vi "Frequency Amplitude Stepped Sweep.vi"(0 "Semiconductor Module Context":T2, 1 "Frequency Sweep (Hz)":dbl[](array[numeric]), 2 "Amplitude Sweep (V)":dbl[](array[numeric]), 5 "Ref Mic Sampling Rate (Hz)":dbl format="%#_13g", 7 "Speaker Sampling Rate (Hz)":dbl format="%#_13g", 11 "error in (no error)":errorcluster) -> (4 "Per-Site Per-Freq Per-Amp dB SPL":dbl[][][](array[numeric]), 15 "error out":errorcluster)   [LabVIEW 2020]
doc: "Frequency Amplitude Stepped Sweep VI returns the Per-Site dB SPL array obtained by sweeping over frequency and amplitude. Also, this VI provides Per-Site TED Bitstream for the passed TSM reference."
uses:
  <vilib>/NI_TestStand_SemiconductorModule/NI_TestStand_Semiconductor_Module.lvlibp/PinMap/General/SemiconductorModuleContext.ctl
  e4dca00a-4e93-4fe6-a22a-85184fe6c6d7.vi
  6f0c4c81-6e94-4ac5-a946-327ae8ed193a.vi
  66372b91-0235-4dd9-a3ee-ceaa2015ee1b.vi
  <vilib>/measure/matone.llb/Extract Single Tone Information N Chan.vi
  <vilib>/NI_TestStand_SemiconductorModule/NI_TestStand_Semiconductor_Module.lvlibp
  <vilib>/measure/NI_MAPro.lvlib
panel:
  in  "Abort":bool
  out "Calibration Progress":dbl(slide) scale=0.0..1.0
  out "Speaker Amplitude":T1(slide)={"Numeric"=0.001, "Numeric"=1.0, "Numeric"=0.001} scale=0.0001..10.0 scale format="%#_6pV"
  out "Frequency":T1(slide)={"Numeric"=100.0, "Numeric"=20000.0, "Numeric"=100.0} scale=10.0..100000.0 scale format="%#_6pHz"
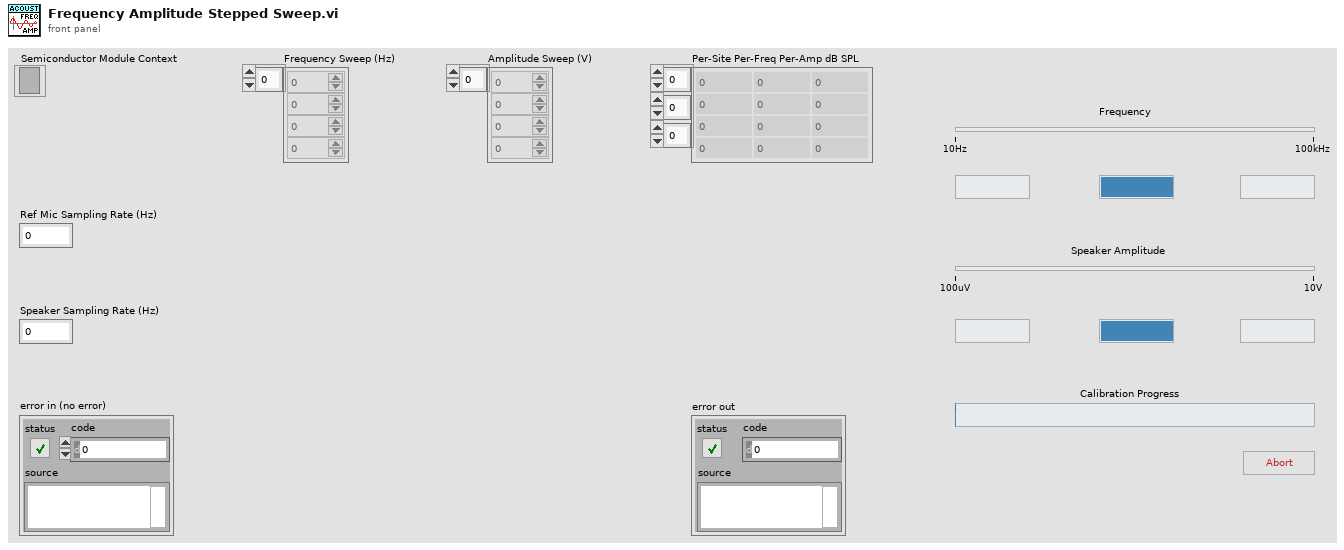
[diagram p1: front panel]
types:
  T1 = cluster{"Numeric":dbl, "Numeric":dbl, "Numeric":dbl}
  T2 = typedef "NI_TestStand_Semiconductor_Module.lvlibp/SemiconductorModuleContext.ctl" = refnum<k7>
  T3 = typedef "TSM DAQmx Multi-Task.ctl" = cluster{"Pin Query Context":refnum<class "MultiplePinMultipleSessionQueryContext.lvclass">, "SSC":T4[], "Site Numbers":i32[], "Pins":tag[]}
  T4 = typedef "SSC DAQmx.ctl" = cluster{"DAQmx Task ":refnum<k21>, "Channels":string, "Channel Lists":string}
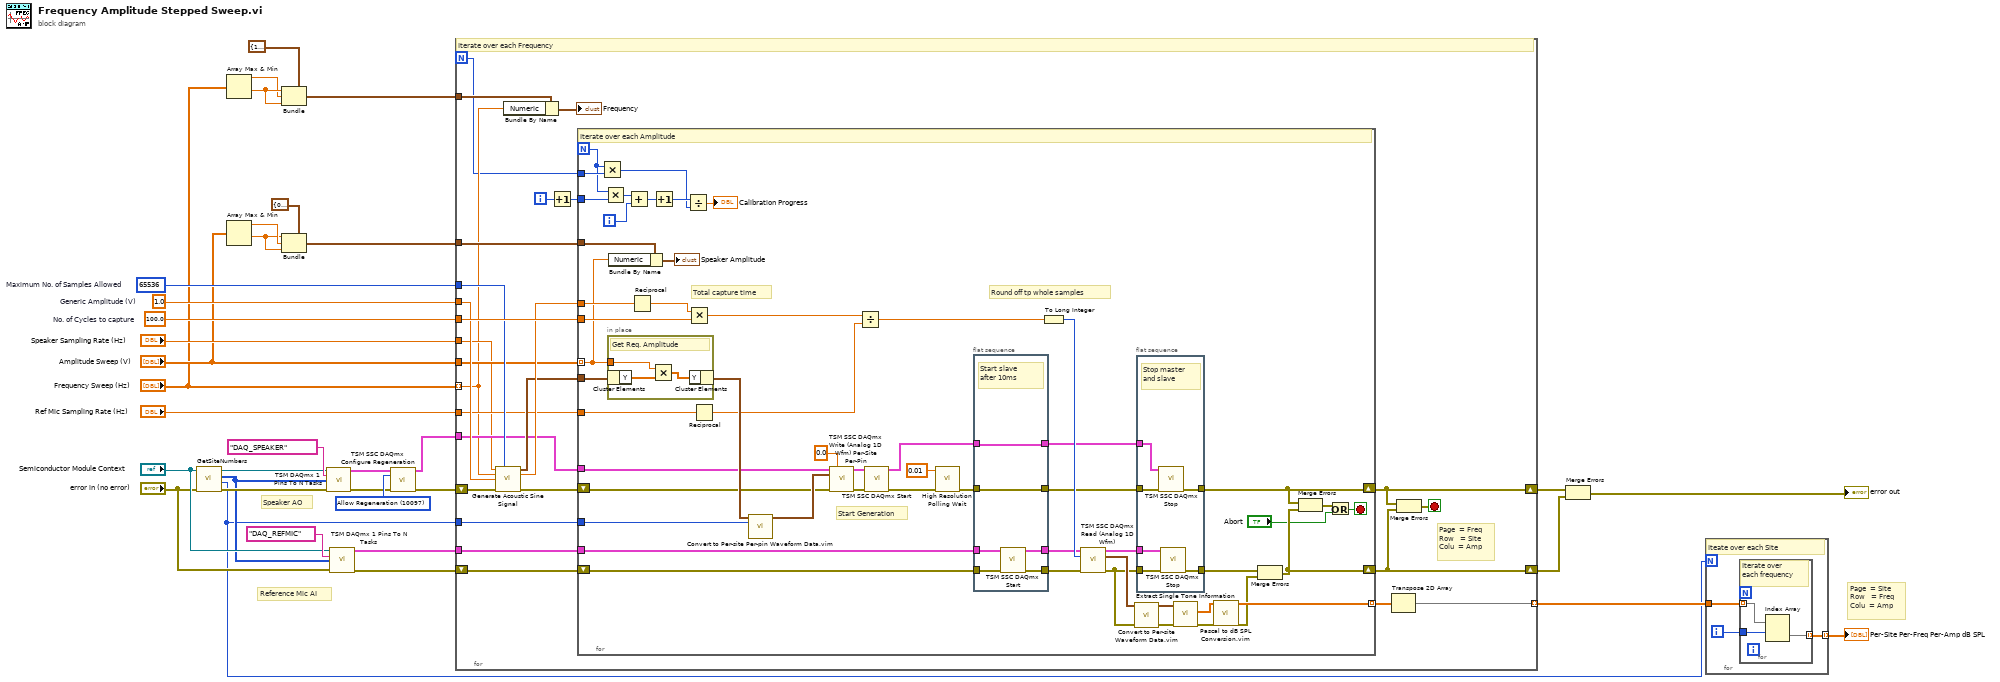
[diagram p0: block diagram]
diagram:
  w15 = 10097 items=["Allow Regeneration"=10097, "Do Not Allow Regeneration"=10158] ("RegenMode")
  w21 = 1.0  # Generic Amplitude (V)
  w26 = 65536  # Maximum No. of Samples Allowed
  w31 = 100.0  # No. of Cycles to capture
  # "Page  = Site\nRow   = Freq\nColu  = Amp"
  # "Reference Mic AI"
  # "Speaker AO"
  n1 = call <vilib>:"GetSiteNumbers.vi"("error in (no error)"="error in (no error)", "Semiconductor Module Context"="Semiconductor Module Context") -> ("error out"=w33:errorcluster, "Number Of Sites"=w19:i32, "Site Numbers"=w25:i32[], "Semiconductor Module Context Out"=w34:T2)  [unwired: 6 in]
  n2 = Array Max & Min(array="Frequency Sweep (Hz)") -> (max value=w6:dbl, min value=w7:dbl)  [unwired: 2 out]
  n3 = Array Max & Min(array="Amplitude Sweep (V)") -> (max value=w9:dbl, min value=w8:dbl)  [unwired: 2 out]
  n4 = Bundle(cluster=T1 {"Numeric"=100.0, "Numeric"=20000.0, "Numeric"=8000.0} ("Frequency"), "Numeric"=w7, "Numeric"=w6, "Numeric"=w7) -> (w4:T1)
  n5 = Bundle(cluster=T1 {"Numeric"=0.001, "Numeric"=1.0, "Numeric"=0.1} ("Speaker Amplitude"), "Numeric"=w8, "Numeric"=w9, "Numeric"=w8) -> (w3:T1)
  n6 = call "TSM DAQmx 1 Pins To N Tasks.vi"("TSM context"=w34, "Pins"=tag "DAQ_SPEAKER", "Site Numbers"=w25, "error in"=w33) -> ("DAQ TSM Out"=w13:T3, "error out"=w14:errorcluster)  [unwired: 10 in]
  n7 = call "TSM DAQmx 1 Pins To N Tasks.vi"("TSM context"="Semiconductor Module Context", "Pins"=tag "DAQ_REFMIC", "Site Numbers"=w25, "error in"="error in (no error)") -> ("DAQ TSM Out"=w22:T3, "error out"=w23:errorcluster)  [unwired: 10 in]
  n8 = call "TSM SSC DAQmx Configure Regeneration.vi"("TSM DAQmx In"=w13, "RegenMode"=w15, "error in (no error)"=w14) -> ("TSM DAQmx Out"=w12:T3, "error out"=w11:errorcluster)  [unwired: 11 in]
  n9 = for {
    N -> [w38]
    shift-right: [w52] -> w30
    shift-left: w11 -> [w61]
    tunnel: "Frequency Sweep (Hz)" -> [w40] mode=indexing
    shift-right: [w51] -> w24
    shift-left: w23 -> [w57]
    tunnel: "Amplitude Sweep (V)" -> [w53]
    tunnel: "Speaker Sampling Rate (Hz)" -> [w43]
    tunnel: w19 -> [w59]
    tunnel: w31 -> [w60]
    tunnel: w26 -> [w58]
    tunnel: w21 -> [w54]
    tunnel: w12 -> [w45]
    tunnel: w22 -> [w56]
    tunnel: [w47] -> w20 mode=indexing
    tunnel: "Ref Mic Sampling Rate (Hz)" -> [w46]
    tunnel: w4 -> [w41]
    tunnel: w3 -> [w42]
    i -> [w37]
    stop <- w50 stop-if-true
    # "Page  = Freq\nRow   = Site\nColu  = Amp"
    # "Iterate over each Frequency"
    n10 = call "Generate Acoustic Sine Signal.vi"("Sampling Rate"=w43, "Maximum No. of Samples Allowed"=w58, "Frequency"=w40, "Sine wave amplitude"=w54, "error in (no error)"=w61) -> ("waveform"=w48:waveform(dbl), "Actual Frequency"=w55:dbl, "error out"=w44:errorcluster)  [unwired: 8 in]
    n11 = Bundle By Name(cluster=w41, "Numeric"=w40) -> (→"Frequency":T1)
    n12 = Increment(x=w37) -> (x+1=w36:i32)
    n13 = for {
      N -> [w69]
      tunnel: w48 -> [w89]
      tunnel: w60 -> [w112]
      tunnel: w59 -> [w105]
      tunnel: w55 -> [w91]
      shift-right: [w82] -> w52
      shift-left: w44 -> [w79]
      shift-right: [w83] -> w51
      shift-left: w57 -> [w99]
      tunnel: w53 -> [w74] mode=indexing
      tunnel: w45 -> [w80]
      tunnel: w56 -> [w98]
      tunnel: [w86] -> w49 mode=indexing
      tunnel: w46 -> [w77]
      tunnel: w42 -> [w75]
      tunnel: w38 -> [w70]
      tunnel: w36 -> [w68]
      i -> [w66]
      stop <- w72 stop-if-true
      # "Start Generation"
      # "Round off tp whole samples"
      # "Total capture time"
      # "Iterate over each Amplitude"
      n14 = Multiply(x=w69, y=w70) -> (x*y=w63:i32)
      n15 = Multiply(x=w69, y=w68) -> (x*y=w67:i32)
      n16 = in-place {
        in-place-border: w74 -> [w116]
        # "Get Req. Amplitude"
        n17 = in-place-cluster #1(w89) -> ("Y"=w115:dbl[])
        n18 = Multiply(x=w116, y=w115) -> (x*y=w114:dbl[])
        n19 = in-place-cluster #1("Y"=w114) -> (w88:waveform(dbl))
      }
      n20 = Bundle By Name(cluster=w75, "Numeric"=w74) -> (→"Speaker Amplitude":T1)
      n21 = Add(x=w67, y=w66) -> (x+y=w65:i32)
      n22 = Reciprocal(x=w91) -> (1/x=w90:dbl)
      n23 = Increment(x=w65) -> (x+1=w64:i32)
      n24 = Divide(x=w64, y=w63) -> (x/y=→"Calibration Progress":dbl)
      n25 = Multiply(x=w90, y=w112) -> (x*y=w103:dbl)
      n26 = Reciprocal(x=w77) -> (1/x=w76:dbl)
      n27 = call "Convert to Per-site Per-pin Waveform Data.vim"("Waveform In"=w88, "No. of Site"=w105) -> ("Per Site Per Pin Waveform Out"=w113:waveform(dbl)[][])  [unwired: 13 in]
      n28 = call "TSM SSC DAQmx Write (Analog 1D Wfm) Per-Site Per-Pin.vi"("DAQ TSM in"=w80, "Idle Channel Value (0)"=0.0, "Per-Site Per-Pin Waveforms in"=w113, "error in"=w79) -> ("DAQ TSM Out"=w111:T3, "error out"=w107:errorcluster)  [unwired: 10 in]
      n29 = Divide(x=w103, y=w76) -> (x/y=w102:dbl)
      n30 = call "TSM SSC DAQmx Start.vi"("TSM DAQmx In"=w111, "error in (no error)"=w107) -> ("TSM DAQmx Out"=w95:T3, "error out"=w104:errorcluster)  [unwired: 12 in]
      n31 = call <vilib>:"High Resolution Polling Wait.vi"("error in (no error)"=w104, "seconds to wait"=0.01) -> ("error out"=w93:errorcluster)  [unwired: 9 in]
      n32 = flat-sequence {
        tunnel: w99 -> [w122]
        tunnel: w98 -> [w121]
        tunnel: [w120] -> w97
        tunnel: [w119] -> w96
        tunnel: w95 -> [w118]
        tunnel: [w118] -> w94
        tunnel: w93 -> [w117]
        tunnel: [w117] -> w92
        frame #0 {
          # "Start slave after 10ms"
          n33 = call "TSM SSC DAQmx Start.vi"("TSM DAQmx In"=w121, "error in (no error)"=w122) -> ("TSM DAQmx Out"=w119:T3, "error out"=w120:errorcluster)  [unwired: 12 in]
        }
      }
      n34 = To Long Integer(number=w102) -> (32bit integer=w101:i32)
      n35 = call "TSM SSC DAQmx Read (Analog 1D Wfm).vi"("DAQ TSM in"=w96, "Samples to read"=w101, "error in"=w97) -> ("DAQ TSM Out"=w110:T3, "Per-Site Per-Pin Waveforms Out"=w109:waveform(dbl)[][], "error out"=w87:errorcluster)  [unwired: 10 in]
      n36 = call "Convert to Per-site Waveform Data.vim"("Per-Site Per-Pin Waveform In"=w109) -> ("Per-Site Waveform Out"=w108:waveform(dbl)[])  [unwired: 14 in]
      n37 = flat-sequence {
        tunnel: w92 -> [w128]
        tunnel: w94 -> [w127]
        tunnel: [w126] -> w82
        tunnel: w87 -> [w125]
        tunnel: [w124] -> w85
        tunnel: w110 -> [w123]
        frame #0 {
          # "Stop master and slave"
          n38 = call "TSM SSC DAQmx Stop.vi"("TSM DAQmx In"=w127, "error in (no error)"=w128) -> ("error out"=w126:errorcluster)  [unwired: 12 in, 1 out]
          n39 = call "TSM SSC DAQmx Stop.vi"("TSM DAQmx In"=w123, "error in (no error)"=w125) -> ("error out"=w124:errorcluster)  [unwired: 12 in, 1 out]
        }
      }
      n40 = call-poly <vilib>:"Extract Single Tone Information.vi"("error in (no error)"=w87, "time signals in"=w108) -> ("error out"=w84:errorcluster, "detected amplitudes"=w78:dbl[])  [unwired: 4 in, 4 out]
      n41 = call "Pascal to dB SPL Conversion.vim"("Pascals"=w78) -> ("dbSPL"=w86:dbl[])  [unwired: 14 in]
      n42 = Merge Errors(w85, w84) -> (w83:errorcluster)
      n43 = Merge Errors(w82, w83) -> (w81:errorcluster)
      n44 = Or(x=w81, y="Abort") -> (x .or. y?=w72:bool)
    }
    n45 = Transpose 2D Array(2D array=w49) -> (transposed array=w47:dbl[][])
    n46 = Merge Errors(w52, w51) -> (w50:errorcluster)
  }
  n47 = Merge Errors(w30, w24) -> (→"error out":errorcluster)
  n48 = for {
    N: w19 -> [_]
    tunnel: w20 -> [w131]
    tunnel: [w129] -> w18 mode=indexing
    i -> [w130]
    # "Iteate over each Site"
    n49 = for {
      tunnel: w131 -> [w134] mode=indexing
      tunnel: w130 -> [w133]
      tunnel: [w132] -> w129 mode=indexing
      # "Iterate over each frequency"
      n50 = Index Array(array=w134, index (row)=w133) -> (element=w132:dbl[])  [unwired: 1 in]
    }
  }
  "Per-Site Per-Freq Per-Amp dB SPL" <- w18
